vi "test Create and Look Into Tx Execution Unit Map.vi"(8 "error in":errorcluster, 11 "TestCase in":refnum<class "Engine.lvclass">) -> (0 "error out":errorcluster, 3 "TestCase out":refnum<class "Engine.lvclass">)   [LabVIEW 2020, in "Engine.lvclass"]
uses:
  Engine.lvclass
  <vilib>/addons/_JKI Toolkits/VI Tester/TestCase.llb/TestCase.lvclass
  <vilib>/NI VeriStand/Custom Device API/Data Reference.ctl
  <vilib>/NI VeriStand/Custom Device API/Custom Device API.lvlib
  <vilib>/NI VeriStand/Custom Device API/Custom Device Item Ref.ctl
  Shared/Transfer Type.ctl
  Encoding and Decoding/Encoding.ctl
  Encoding and Decoding/Encoding and Decoding.lvlib
  Shared/Parameter Definition.ctl
  Shared/RT Parameters.ctl
  Shared/Label.ctl
  Shared/RT Label Settings.ctl
  Shared/RT Hardware Channel Settings.ctl
  Engine/Custom Device/Custom Device.lvlib
  C:/Program Files (x86)/National Instruments/LabVIEW 2020/vi.lib/addons/_JKI Toolkits/VI Tester/TestCase.llb/TestCase.lvclass
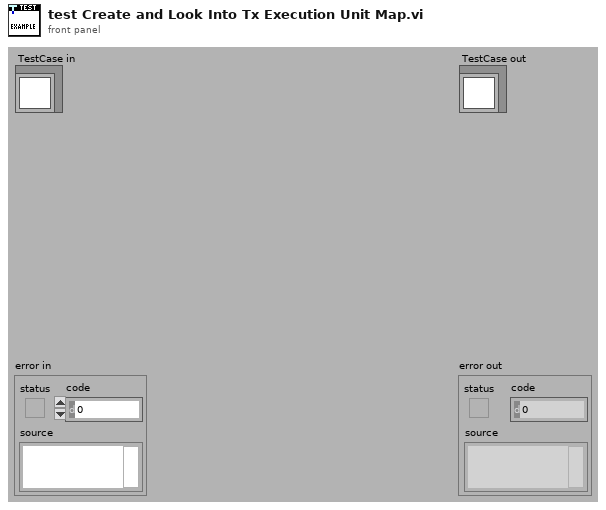
[diagram p1: front panel]
types:
  T1 = typedef "RT Hardware Channel Settings.ctl" = cluster{"channel #":u16, "channel handle":u64, "labels settings for RT":T2[]}
  T2 = typedef "RT Label Settings.ctl" = cluster{"Name":string, "xmlName":string, "label":T3, "transfer period":u32, "SDI_Enabled":bool, "SDI":u8, "parameter driver data":T4, "transfer type":T8, "has timestamp?":bool, "Label Disable/Trigger Channel Reference":T7, "Message Handle":u64, "Initialized?":bool, "Word Initial Raw Value":u32, "Label Timestamp Channel Data Reference":T9, "disabled":bool}
  T3 = typedef "Label.ctl" = u8
  T4 = typedef "RT Parameters.ctl" = cluster{"parameter definitions":T5[], "Tx parameter refs":T7[]}
  T5 = typedef "Parameter Definition.ctl" = cluster{"start index":i32, "size":i32, "encoding":T6, "signed":bool, "scale multiplier":dbl, "scale offset":dbl}
  T6 = typedef "Encoding and Decoding.lvlib/Encoding.ctl" = enum16{"BNR", "BCD", "Discrete"}
  T7 = typedef "Custom Device API.lvlib/Custom Device Item Ref.ctl" = u64
  T8 = typedef "Transfer Type.ctl" = enum16{"Scheduled", "Acyclic", "Block", "Strobe"}
  T9 = typedef "Custom Device API.lvlib/Data Reference.ctl" = i32
  T10 = cluster{"channel index":i32, "label index":i32, "group values start index":i32, "values in group":i32}
  T11 = typedef "Map of Values Indexes to Channel and Label Indexes.ctl" = map{i32, cluster{"channel index":i32, "label index":i32, "group values start index":i32, "values in group":i32}}
  T12 = cluster{"channel index":i32, "label index":i32, "group values start index":i32, "values in group":i32}[]
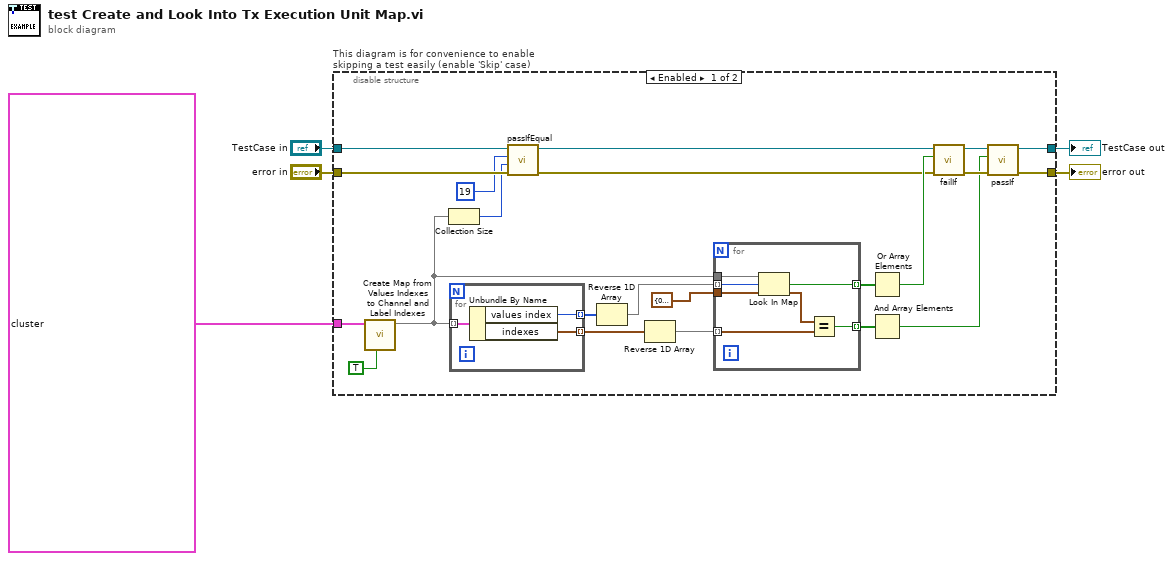
[diagram p0: block diagram]
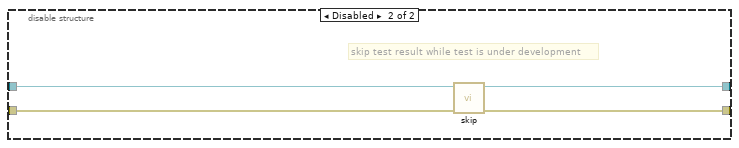
[diagram p2: hidden frame]
diagram:
  n1 = disable-structure "This diagram is for convenience to enable skipping a test easily (enable 'Skip' case)" shown="Enabled" {
    disable-tunnel: "TestCase in" -> [w11 w41]
    disable-tunnel: [w27 w39] -> w2
    disable-tunnel: [w26 w40] -> w4
    disable-tunnel: "error in" -> [w10 w38]
    disable-tunnel: T1[] [{"channel #"=0, "channel handle"=0, "labels settings for RT"=[]}, {"channel #"=1, "channel handle"=0, "labels settings for RT"=[{"Name"="", "xmlName"="", "label"=11, "transfer period"=0, "SDI_Enabled"=FALSE, "SDI"=0, "parameter driver data"={"parameter definitions"=[{"start index"=10, "size"=16, "encoding"=enum."BCD", "signed"=TRUE, "scale multiplier"=1.0, "scale offset"=0.0}], "Tx parameter refs"=[]}, "transfer type"=enum."Scheduled", "has timestamp?"=TRUE, "Label Disable/Trigger Channel Reference"=0, "Message Handle"=0, "Initialized?"=TRUE, "Word Initial Raw Value"=0, "Label Timestamp Channel Data Reference"=0, "disabled"=FALSE}]}, {"channel #"=0, "channel handle"=0, "labels settings for RT"=[]}, {"channel #"=3, "channel handle"=0, "labels settings for RT"=[{"Name"="", "xmlName"="", "label"=33, "transfer period"=0, "SDI_Enabled"=FALSE, "SDI"=0, "parameter driver data"={"parameter definitions"=[{"start index"=10, "size"=19, "encoding"=enum."BNR", "signed"=TRUE, "scale multiplier"=0.0, "scale offset"=0.0}], "Tx parameter refs"=[]}, "transfer type"=enum."Scheduled", "has timestamp?"=FALSE, "Label Disable/Trigger Channel Reference"=0, "Message Handle"=0, "Initialized?"=TRUE, "Word Initial Raw Value"=0, "Label Timestamp Channel Data Reference"=0, "disabled"=FALSE}]}, {"channel #"=0, "channel handle"=0, "labels settings for RT"=[]}, {"channel #"=5, "channel handle"=0, "labels settings for RT"=[{"Name"="", "xmlName"="", "label"=55, "transfer period"=0, "SDI_Enabled"=FALSE, "SDI"=0, "parameter driver data"={"parameter definitions"=[{"start index"=10, "size"=3, "encoding"=enum."BCD", "signed"=FALSE, "scale multiplier"=0.0, "scale offset"=0.0}, {"start index"=13, "size"=4, "encoding"=enum."BCD", "signed"=FALSE, "scale multiplier"=0.0, "scale offset"=0.0}, {"start index"=17, "size"=4, "encoding"=enum."BCD", "signed"=FALSE, "scale multiplier"=0.0, "scale offset"=0.0}, {"start index"=21, "size"=4, "encoding"=enum."BCD", "signed"=FALSE, "scale multiplier"=0.0, "scale offset"=0.0}, {"start index"=25, "size"=4, "encoding"=enum."BCD", "signed"=FALSE, "scale multiplier"=0.0, "scale offset"=0.0}], "Tx parameter refs"=[]}, "transfer type"=enum."Scheduled", "has timestamp?"=FALSE, "Label Disable/Trigger Channel Reference"=0, "Message Handle"=0, "Initialized?"=TRUE, "Word Initial Raw Value"=0, "Label Timestamp Channel Data Reference"=0, "disabled"=FALSE}]}, {"channel #"=0, "channel handle"=0, "labels settings for RT"=[]}, {"channel #"=0, "channel handle"=0, "labels settings for RT"=[]}, {"channel #"=0, "channel handle"=0, "labels settings for RT"=[]}, {"channel #"=0, "channel handle"=0, "labels settings for RT"=[]}, {"channel #"=0, "channel handle"=0, "labels settings for RT"=[]}, {"channel #"=0, "channel handle"=0, "labels settings for RT"=[]}, {"channel #"=0, "channel handle"=0, "labels settings for RT"=[]}, {"channel #"=0, "channel handle"=0, "labels settings for RT"=[]}, {"channel #"=0, "channel handle"=0, "labels settings for RT"=[]}, {"channel #"=15, "channel handle"=0, "labels settings for RT"=[{"Name"="", "xmlName"="", "label"=155, "transfer period"=0, "SDI_Enabled"=FALSE, "SDI"=0, "parameter driver data"={"parameter definitions"=[{"start index"=10, "size"=1, "encoding"=enum."Discrete", "signed"=FALSE, "scale multiplier"=0.0, "scale offset"=0.0}, {"start index"=11, "size"=1, "encoding"=enum."Discrete", "signed"=FALSE, "scale multiplier"=0.0, "scale offset"=0.0}, {"start index"=12, "size"=1, "encoding"=enum."Discrete", "signed"=FALSE, "scale multiplier"=0.0, "scale offset"=0.0}, {"start index"=13, "size"=1, "encoding"=enum."Discrete", "signed"=FALSE, "scale multiplier"=0.0, "scale offset"=0.0}, {"start index"=14, "size"=1, "encoding"=enum."Discrete", "signed"=FALSE, "scale multiplier"=0.0, "scale offset"=0.0}], "Tx parameter refs"=[]}, "transfer type"=enum."Scheduled", "has timestamp?"=FALSE, "Label Disable/Trigger Channel Reference"=0, "Message Handle"=0, "Initialized?"=TRUE, "Word Initial Raw Value"=0, "Label Timestamp Channel Data Reference"=0, "disabled"=FALSE}]}, {"channel #"=0, "channel handle"=0, "labels settings for RT"=[]}, {"channel #"=0, "channel handle"=0, "labels settings for RT"=[]}, {"channel #"=0, "channel handle"=0, "labels settings for RT"=[]}, {"channel #"=0, "channel handle"=0, "labels settings for RT"=[]}, {"channel #"=0, "channel handle"=0, "labels settings for RT"=[]}, {"channel #"=0, "channel handle"=0, "labels settings for RT"=[]}, {"channel #"=0, "channel handle"=0, "labels settings for RT"=[]}, {"channel #"=0, "channel handle"=0, "labels settings for RT"=[]}, {"channel #"=0, "channel handle"=0, "labels settings for RT"=[]}, {"channel #"=25, "channel handle"=0, "labels settings for RT"=[{"Name"="", "xmlName"="", "label"=255, "transfer period"=0, "SDI_Enabled"=FALSE, "SDI"=0, "parameter driver data"={"parameter definitions"=[{"start index"=0, "size"=0, "encoding"=enum."BNR", "signed"=FALSE, "scale multiplier"=0.0, "scale offset"=0.0}], "Tx parameter refs"=[]}, "transfer type"=enum."Scheduled", "has timestamp?"=FALSE, "Label Disable/Trigger Channel Reference"=0, "Message Handle"=0, "Initialized?"=TRUE, "Word Initial Raw Value"=0, "Label Timestamp Channel Data Reference"=0, "disabled"=FALSE}]}, {"channel #"=0, "channel handle"=0, "labels settings for RT"=[]}, {"channel #"=0, "channel handle"=0, "labels settings for RT"=[]}, {"channel #"=0, "channel handle"=0, "labels settings for RT"=[]}, {"channel #"=0, "channel handle"=0, "labels settings for RT"=[]}, {"channel #"=0, "channel handle"=0, "labels settings for RT"=[]}, {"channel #"=0, "channel handle"=0, "labels settings for RT"=[{"Name"="", "xmlName"="", "label"=0, "transfer period"=0, "SDI_Enabled"=FALSE, "SDI"=0, "parameter driver data"={"parameter definitions"=[], "Tx parameter refs"=[]}, "transfer type"=enum."Scheduled", "has timestamp?"=FALSE, "Label Disable/Trigger Channel Reference"=0, "Message Handle"=0, "Initialized?"=FALSE, "Word Initial Raw Value"=0, "Label Timestamp Channel Data Reference"=0, "disabled"=FALSE}]}] ("RT hardware channel data") -> [w25 _]
    frame Enabled {
      n2 = call "Create Map from Values Indexes to Channel and Label Indexes.vi"("disable channel included in group"=TRUE, "RT hardware channels"=w25) -> ("map from values index to RT info indexes"=w14:T11)  [unwired: 8 in, 1 out]
      n3 = Collection Size(1:w14) -> (0:w9:i32)
      n4 = for {
        tunnel: w14 -> [w37] mode=indexing
        tunnel: [w36] -> w24 mode=indexing
        tunnel: [w35] -> w23 mode=indexing
        n5 = Unbundle By Name(w37) -> ("values index"=w36:i32, "indexes"=w35:T10)
      }
      n6 = call-dynamic "passIfEqual.vi"("error in (no error)"=w10, "y"=w9, "x"=19 ("size"), "TestCase in"=w11) -> ("error out"=w12:errorcluster, "TestCase out"=w13:refnum<class "Engine.lvclass">)  [unwired: 6 in]
      n7 = Reverse 1D Array(array=w24) -> (reversed array=w22:i32[])
      n8 = Reverse 1D Array(array=w23) -> (reversed array=w17:T12)
      n9 = for {
        tunnel: w14 -> [w34]
        tunnel: w22 -> [w33] mode=indexing
        tunnel: [w32] -> w21 mode=indexing
        tunnel: w17 -> [w30] mode=indexing
        tunnel: [w29] -> w16 mode=indexing
        tunnel: T10 {"channel index"=0, "label index"=0, "group values start index"=0, "values in group"=0} ("default value") -> [w28]
        n10 = Look In Map(map=w34, key=w33, default value=w28) -> (key not found?=w32:bool, value=w31:T10)
        n11 = Equal?(x=w31, y=w30) -> (x = y?=w29:bool)
      }
      n12 = Or Array Elements(Boolean array=w21) -> (logical OR=w20:bool)
      n13 = And Array Elements(Boolean array=w16) -> (logical AND=w15:bool)
      n14 = call-dynamic "failIf.vi"("error in (no error)"=w12, "fail"=w20, "TestCase in"=w13) -> ("error out"=w18:errorcluster, "TestCase out"=w19:refnum<class "Engine.lvclass">)  [unwired: 7 in]
      n15 = call-dynamic "passIf.vi"("error in (no error)"=w18, "pass"=w15, "TestCase in"=w19) -> ("error out"=w26:errorcluster, "TestCase out"=w27:refnum<class "Engine.lvclass">)  [unwired: 7 in]
    }
    frame Disabled {
      # "skip test result while test is under development"
      n16 = call <vilib>:"skip.vi"("error in (no error)"=w38, "TestCase in"=w41) -> ("error out"=w40:errorcluster, "TestCase out"=w39:refnum<class "Engine.lvclass">)  [unwired: 8 in]
    }
  }
  "error out" <- w4
  "TestCase out" <- w2
